vi "Read Worker Type.vi"(8 "error in (no error)":errorcluster, 11 "Worker in":refnum<class "Worker.lvclass">) -> (0 "error out":errorcluster, 2 "Type":string, 3 "Worker out":refnum<class "Worker.lvclass">)   [LabVIEW 2023, in "Worker.lvlib" / "Worker.lvclass"]
doc: "Returns the type of worker. This method is required by any descendant of the Worker class."
uses:
  Worker.lvclass
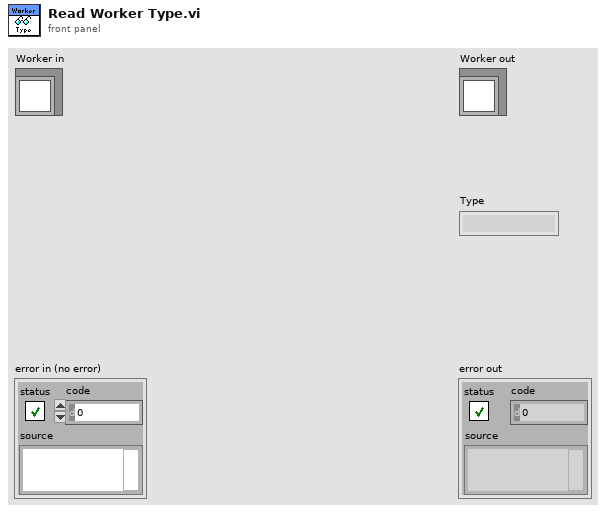
[diagram p1: front panel]
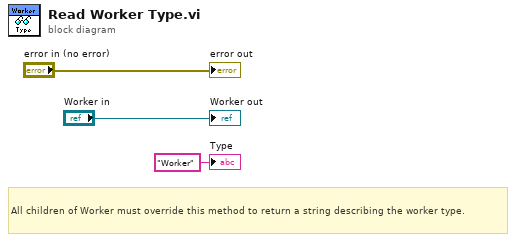
[diagram p0: block diagram]
diagram:
  # "All children of Worker must override this method to return a string describing the worker type."
  "error out" <- "error in (no error)"
  "Worker out" <- "Worker in"
  "Type" <- "Worker" ("Type")
